vi "finish_position.vi"(5 "finish_position":bool, 7 "end_experiment":bool=TRUE, 8 "error in (no error)":errorcluster, 11 "Stage IN":refnum<class "Stage.lvclass">) -> (0 "error out":errorcluster, 3 "Stage out 2":refnum<class "Stage.lvclass">)   [LabVIEW 2015, in "pcfs.lvclass"]
uses:
  pcfs.lvclass
  Stage Class/Stage.lvclass
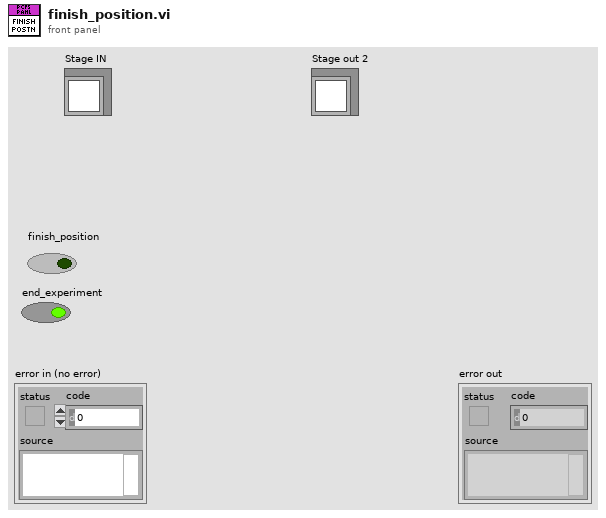
[diagram p1: front panel]
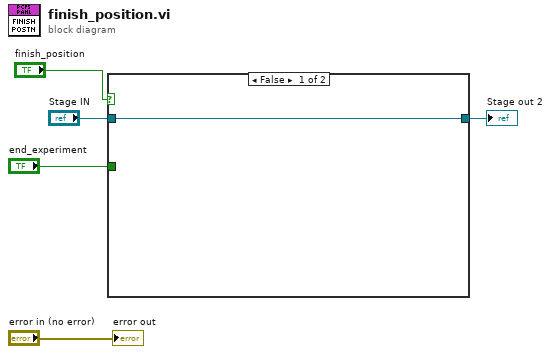
[diagram p0: block diagram]
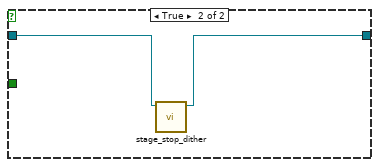
[diagram p2: hidden frame]
diagram:
  n1 = case shown="False" "finish_position" {
    tunnel: "Stage IN" -> [w6 w8]
    tunnel: [w6 w7] -> w3
    tunnel: "end_experiment" -> [_ _]
    frame False {
    }
    frame True {
      n2 = call-dynamic "stage_stop_dither.vi"("Stage in"=w8) -> ("Stage out"=w7:refnum<class "Stage.lvclass">)  [unwired: 9 in, 1 out]
    }
  }
  "Stage out 2" <- w3
  "error out" <- "error in (no error)"
